vi "runscenario retrieve Files.vi"(8 "error in (no error)":errorcluster, 9 "exportContent (\"\")":string, 10 "filename (\"\": use POST)":string, 11 "sxScenarioId (\"\")":string) -> (0 "error out":errorcluster, 1 "Filename":string, 2 "Content":string)   [LabVIEW 2011]
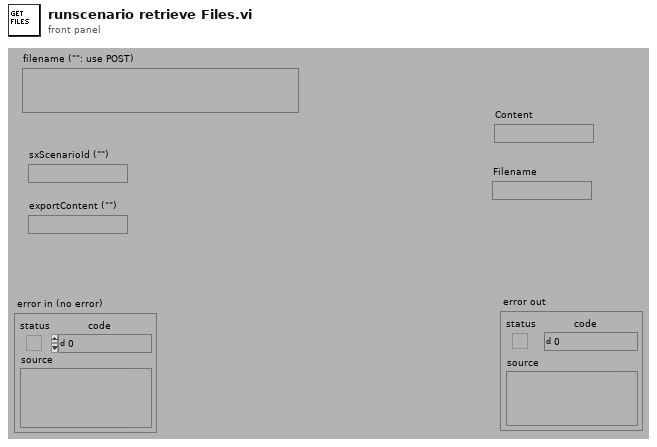
[diagram p1: front panel]
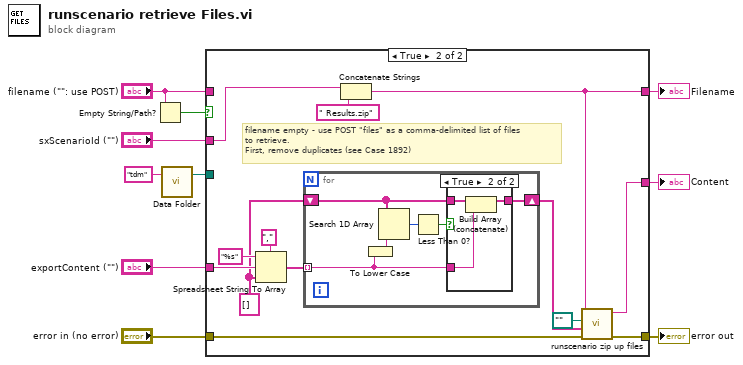
[diagram p0: block diagram]
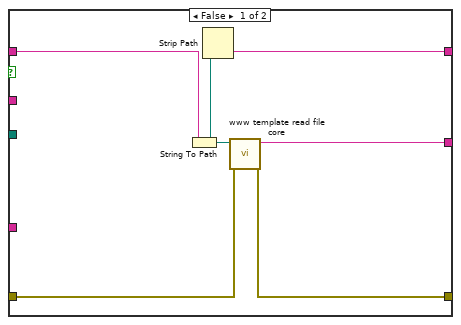
[diagram p2: hidden frame]
diagram:
  n1 = Empty String/Path?(string/path="filename (\"\": use POST)") -> (empty?=w8:bool)
  n2 = call "Data Folder.vi"("Relative Path (\"\" - Folder)"="tdm" ("Relative Path (\"\" - Folder)")) -> ("Data Folder"=w5:path)  [unwired: 2 in]
  n3 = case shown="True" w8 {
    tunnel: [w11 w18] -> w10
    tunnel: "exportContent (\"\")" -> [_ w24]
    tunnel: "filename (\"\": use POST)" -> [w12 _]
    tunnel: w5 -> [_ _]
    tunnel: "error in (no error)" -> [w16 w27]
    tunnel: [w15 w25] -> w3
    tunnel: [w14 w26] -> w2
    tunnel: "sxScenarioId (\"\")" -> [_ w19]
    frame False {
      n4 = String To Path(string=w12) -> (path=w13:path)
      n5 = Strip Path(path=w13) -> (name=w11:string)  [unwired: 1 out]
      n6 = call "www template read file core.vi"("error in (no error)"=w16, "Path"=w13) -> ("error out"=w15:errorcluster, "File Content"=w14:string)  [unwired: 8 out]
    }
    frame True {
      w22 = string[] []
      # "filename empty - use POST \"files\" as a comma-delimited list of files\nto retrieve.\nFirst, remove duplicates (see Case 1892)"
      n7 = Spreadsheet String To Array(delimiter (Tab)=",", format string="%s" ("Template (\"\")"), spreadsheet string=w24, array type (2D Dbl)=w22) -> (array=w23:string[])
      n8 = for {
        tunnel: w23 -> [w30] mode=indexing
        shift-right: [w32] -> w21
        shift-left: w22 -> [w33]
        n9 = To Lower Case(string=w30) -> (all lower case string=w31:string)
        n10 = Search 1D Array(1D array=w33, element=w31) -> (index of element=w35:i32)  [unwired: 1 in]
        n11 = Less Than 0?(x=w35) -> (x < 0?=w34:bool)
        n12 = case shown="True" w34 {
          tunnel: w33 -> [w36 w39]
          tunnel: [w36 w38] -> w32
          tunnel: w30 -> [_ w37]
          frame False {
          }
          frame True {
            n13 = Build Array (concatenate)(w39, w37) -> (w38:string[])
          }
        }
      }
      n14 = Concatenate Strings(w19, " Results.zip" ("Template (\"\")")) -> (w18:string)
      n15 = call "runscenario zip up files.vi"("error in (no error)"=w27, "Filenames to Zip (empty)"=w21, "Path to Files (empty)"=path "", "Zip filename (\"\")"=w18) -> ("error out"=w25:errorcluster, "Content"=w26:string)  [unwired: 6 out]
    }
  }
  "error out" <- w3
  "Content" <- w2
  "Filename" <- w10
